vi "data.vi"() -> ()   [LabVIEW 2016]
uses:
  <vilib>/dex/Stream Element Allocation Mode.ctl
panel:
  in  "Lenkung":dbl(slide) scale=-110.0..110.0
  in  "stop":bool
  in  "schpeed":dbl(knob)=0.5 scale=0.2..0.4
  # "GAS"
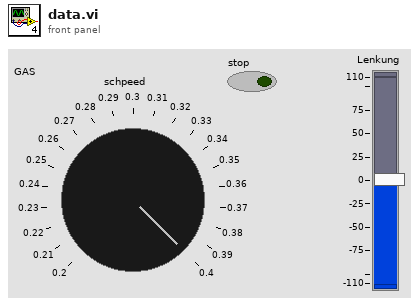
[diagram p1: front panel]
types:
  T1 = typedef "Stream Element Allocation Mode.ctl" = u32
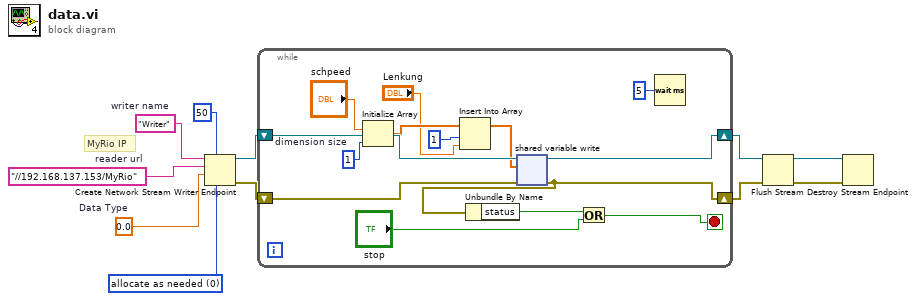
[diagram p0: block diagram]
diagram:
  w4 = T1 0 items=["allocate as needed", "pre-allocate"] ("element allocation mode")
  w5 = "//192.168.137.153/MyRio"  # reader url
  w10 = "Writer"  # writer name
  w11 = 0.0  # Data Type
  # "MyRio IP"
  n1 = Create Network Stream Writer Endpoint(6:w4, 7:50 ("writer buffer size"), 9:w11, 10:w5, 11:w10) -> (0:w9:errorcluster, 3:w8:refnum<k21>)  [unwired: 2 in]
  n2 = while {
    shift-right: [w13] -> w1
    shift-left: w8 -> [w24]
    shift-right: [w12] -> w2
    shift-left: w9 -> [w25]
    stop <- w22 stop-if-true
    w19 = 1  # dimension size
    n3 = Initialize Array("schpeed", w19) -> (w18:dbl[])
    n4 = Insert Into Array(array=w18, index=1, new element="Lenkung") -> (w14:dbl[])
    n5 = shared-variable-write ("Write Multiple Elements to Stream")(w24, w25, w14) -> (w13:refnum<k21>, w12:errorcluster)  [unwired: 1 in, 1 out]
    n6 = Unbundle By Name "Unbundle By Name"(w12) -> ("status"=w23:bool)
    n7 = Or(x=w23, y="stop") -> (x .or. y?=w22:bool)
    n8 = Wait (ms)(milliseconds to wait=u32 5) -> ()  [unwired: 1 out]
  }
  n9 = Flush Stream(8:w2, 11:w1) -> (0:w7:errorcluster, 3:w6:refnum<k21>)  [unwired: 2 in, 1 out]
  n10 = Destroy Stream Endpoint(8:w7, 11:w6) -> ()  [unwired: 1 out]
